vi "ReadLightTower&SwitchStatus.vi"(0 "UDP Network Connection in":refnum<k16>, 1 "IP Address of SNMP Device":string, 2 "RoomAlert in":refnum<class "RoomAlert.lvclass">, 5 "Community Name":string, 7 "Array In":waveform(dbl)[](array[waveform]), 9 "Timeout(ms)":i32, 11 "error in (no error)":errorcluster, 12 "LightTower OID":string[][](array[string]), 13 "Amber Warning Light Limits":T1) -> (4 "Light Tower":T2, 8 "Array Out":waveform(dbl)[](array[waveform]), 10 "Yellow Limit Exceeded?":bool, 15 "error out":errorcluster)   [LabVIEW 2018, in "SensorPlugins.lvlib" / "RoomAlert.lvclass"]
doc: "Reads the Light Tower and Switch Sensor status"
uses:
  RoomAlert.lvclass
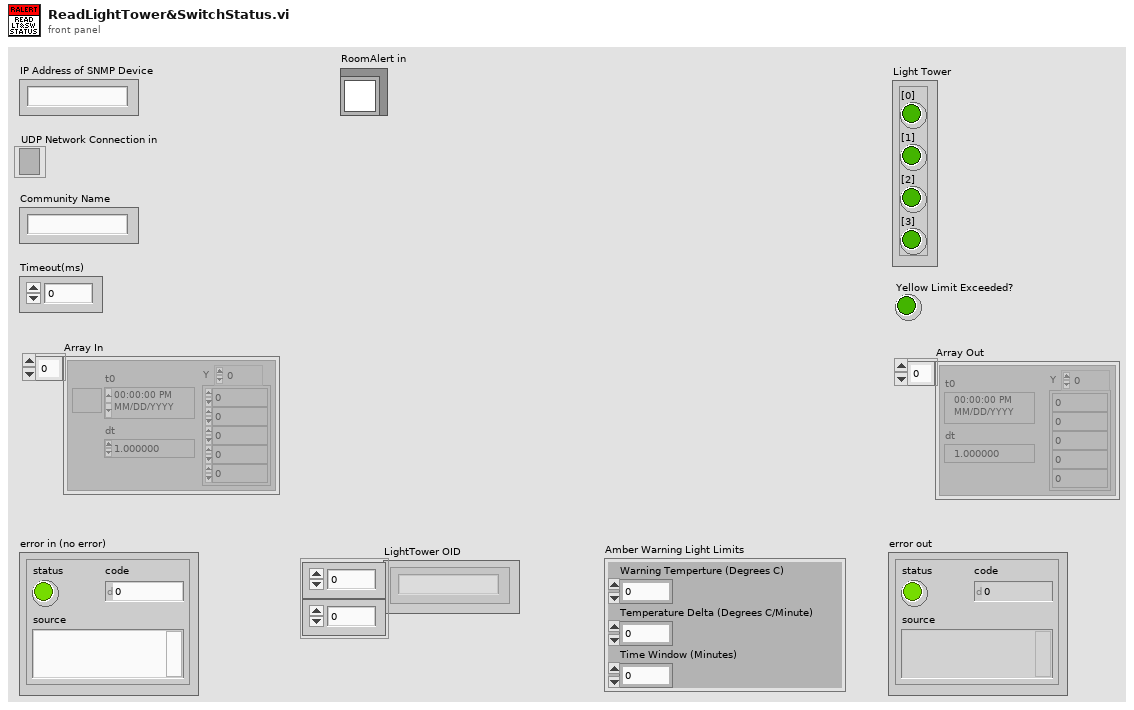
[diagram p1: front panel]
types:
  T1 = cluster{"Warning Temperture (Degrees C)":dbl, "Temperature Delta (Degrees C/Minute)":dbl, "Time Window (Minutes)":dbl}
  T2 = cluster{"[0]":bool, "[1]":bool, "[2]":bool, "[3]":bool}
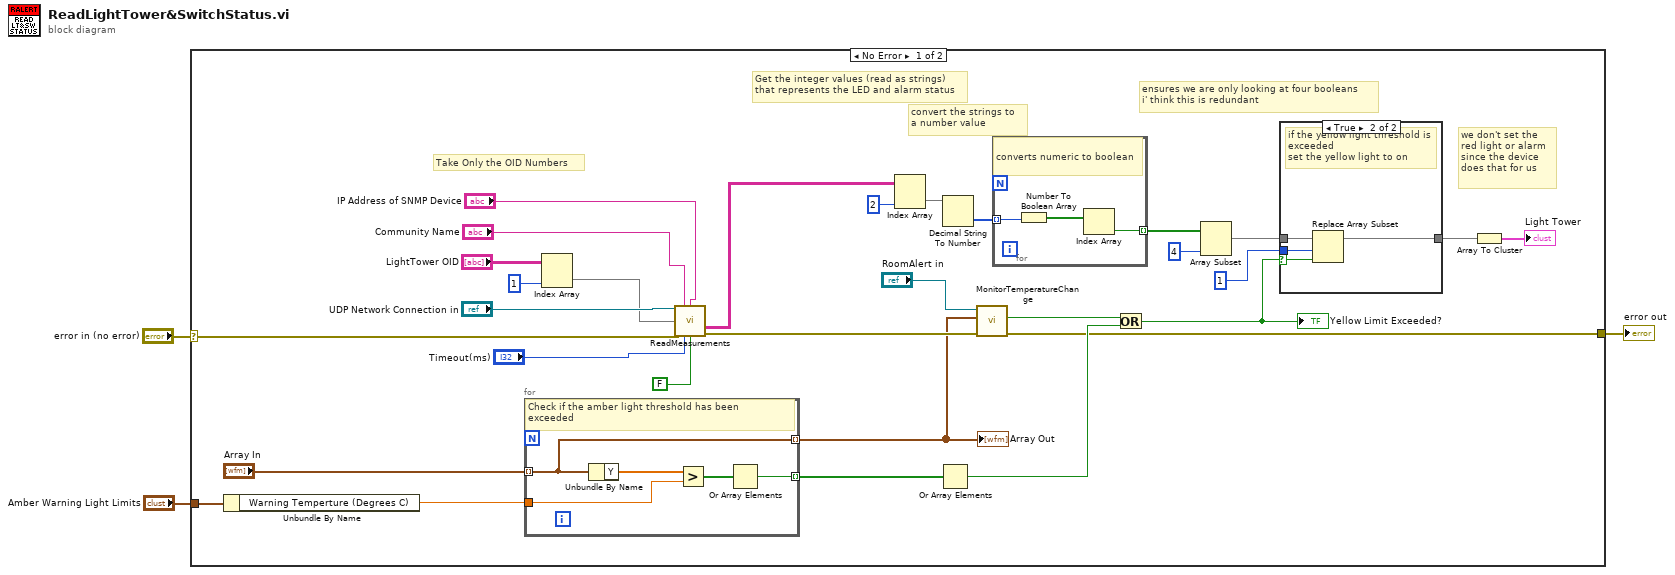
[diagram p0: block diagram]
diagram:
  n1 = case shown="No Error" "error in (no error)" {
    selector: "error in (no error)" -> [w12 w47]
    tunnel: [w17 w47] -> w2
    tunnel: "Amber Warning Light Limits" -> [w22 _]
    frame No Error {
      # "we don't set the \nred light or alarm \nsince the device \ndoes that for us"
      # "ensures we are only looking at four booleans\ni' think this is redundant"
      # "convert the strings to \na number value"
      # "Get the integer values (read as strings)\nthat represents the LED and alarm status"
      # "Take Only the OID Numbers"
      n2 = Unbundle By Name(w22) -> ("Warning Temperture (Degrees C)"=w21:dbl)
      n3 = for {
        tunnel: "Array In" -> [w39] mode=indexing
        tunnel: [w41] -> w26 mode=indexing
        tunnel: w21 -> [w40]
        tunnel: [w39] -> w15 mode=indexing
        # "Check if the amber light threshold has been\nexceeded"
        n4 = Unbundle By Name(w39) -> ("Y"=w43:dbl[])
        n5 = Greater?(x=w43, y=w40) -> (0:w42:bool[])
        n6 = Or Array Elements(Boolean array=w42) -> (logical OR=w41:bool)
      }
      "Array Out" <- w15
      n7 = Index Array(array="LightTower OID", index (col)=1 ("disabled index (col)")) -> (element=w8:string[])  [unwired: 1 in]
      n8 = call "ReadMeasurements.vi"("UDP Network Connection in"="UDP Network Connection in", "Community Name"="Community Name", "IP Address of SNMP Device"="IP Address of SNMP Device", "OID Numbers"=w8, "error in (no error)"=w12, "Timeout(ms)"="Timeout(ms)", "Filter OID Numbers? (T)"=FALSE) -> ("SNMPDataAsStrings"=w6:string[][], "error out"=w18:errorcluster)  [unwired: 6 in, 1 out]
      n9 = Index Array(array=w6, index (col)=2 ("disabled index (col)")) -> (element=w31:string[])  [unwired: 1 in]
      n10 = Or Array Elements(Boolean array=w26) -> (logical OR=w20:bool)
      n11 = Decimal String To Number(string=w31) -> (number=w30:i32[])  [unwired: 2 in, 1 out]
      n12 = call-dynamic "MonitorTemperatureChange.vi"("error in (no error)"=w18, "Array Out"=w15, "RoomAlert in"="RoomAlert in") -> ("error out"=w17:errorcluster, "TempChangeExceedLimits"=w19:bool)  [unwired: 6 in, 1 out]
      n13 = for {
        tunnel: w30 -> [w45] mode=indexing
        tunnel: [w44] -> w29 mode=indexing
        # "converts numeric to boolean"
        n14 = Number To Boolean Array(number=w45) -> (Boolean array=w46:bool[])
        n15 = Index Array(array=w46) -> (element=w44:bool)  [unwired: 1 in]
      }
      n16 = Or(x=w19, y=w20) -> (x .or. y?=w14:bool)
      "Yellow Limit Exceeded?" <- w14
      n17 = Array Subset(array=w29, length=4) -> (w25:bool[])  [unwired: 1 in]
      n18 = case shown="True" w14 {
        selector: w14 -> [_ w35]
        tunnel: w25 -> [w34 w38]
        tunnel: 1 ("index") -> [_ w37]
        tunnel: [w34 w36] -> w23
        frame False {
        }
        frame True {
          # "if the yellow light threshold is exceeded \nset the yellow light to on"
          n19 = Replace Array Subset(array=w38, new element=w35, index=w37) -> (w36:bool[])
        }
      }
      n20 = Array To Cluster(array=w23) -> (cluster=→"Light Tower":T2)
    }
    frame Error {
    }
  }
  "error out" <- w2
